vi "Zamojski_prac8.vi"() -> ()   [LabVIEW 2020]
uses:
  <vilib>/Platform/TimedLoop/XDataNode/timing_clust.ctl
  <vilib>/Platform/TimedLoop/XDataNode/nitl_modes.ctl
  <vilib>/Platform/TimedLoop/XDataNode/wakeup.ctl
  <vilib>/Platform/TimedLoop/scheduler/LVUserAPI/_suppVIs/Create_1kHz_TSource.vi
  <vilib>/platform/TimedLoop/XDataNode/XDataNode.xnode
  <vilib>/Platform/TimedLoop/XDataNode/XDNodeRunTimeDep.lvlib
panel:
  out "L2 Error":errorcluster
  out "czas_pocz_L1":dbl
  out "L1 Error":errorcluster
  out "L1 Iteracja":dbl
  out "L2 Koniec":bool
  out "L1 Koniec":bool
  out "L2 Stop":dbl
  out "L2 End":dbl
  out "L1 Stop":dbl
  out "L1 End":dbl
  out "L2 Iteracja":dbl
  out "SO End":dbl
  out "SO Start":dbl
  in  "Synchronizacja":bool
  in  "Okres (s)":dbl=0.5 min=0.5 max=20.0 step=0.5
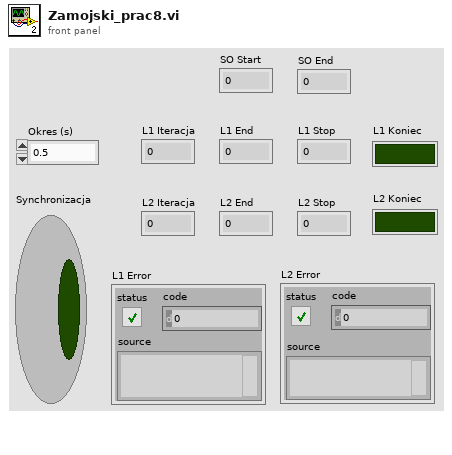
[diagram p1: front panel]
types:
  T1 = typedef "XDNodeRunTimeDep.lvlib/timing_clust.ctl" = cluster{"Expected End [f-1]":u64, "Actual End [f-1]":u64, "Finished Late? [f-1]":bool, "Expected End [i-1]":u64, "Actual End [i-1]":u64, "Finished Late? [i-1]":bool, "Expected Start [i]":u64, "Actual Start [i]":u64, "Expected Start [f]":u64, "Actual Start [f]":u64, "Source Name":string, "Structure Name":string, "Period":i64, "Deadline":i64, "Offset":i64, "Start":i64, "Priority":i32, "Timeout":i32, "Mode":T2, "Wakeup Reason":T3, "Error":errorcluster, "Source Type":string, "Secondary Source Type":string, "Global End Time":u64, "Global Start Time":u64, "Frame Duration":u64, "Iteration Duration":u64, "Assigned CPU":i32, "I/O Scan Engine Mode":u32}
  T2 = typedef "XDNodeRunTimeDep.lvlib/nitl_modes.ctl" = enum32{"No Change", "Process missed periods, maintain original phase", "Discard missed periods, maintain original phase", "Process missed periods, ignore original phase", "Discard missed periods, ignore original phase"}
  T3 = typedef "XDNodeRunTimeDep.lvlib/wakeup.ctl" = enum32{"Normal", "Aborted", "Asynchronous wakeup", "Timing source error", "Timed loop error", "Timeout"}
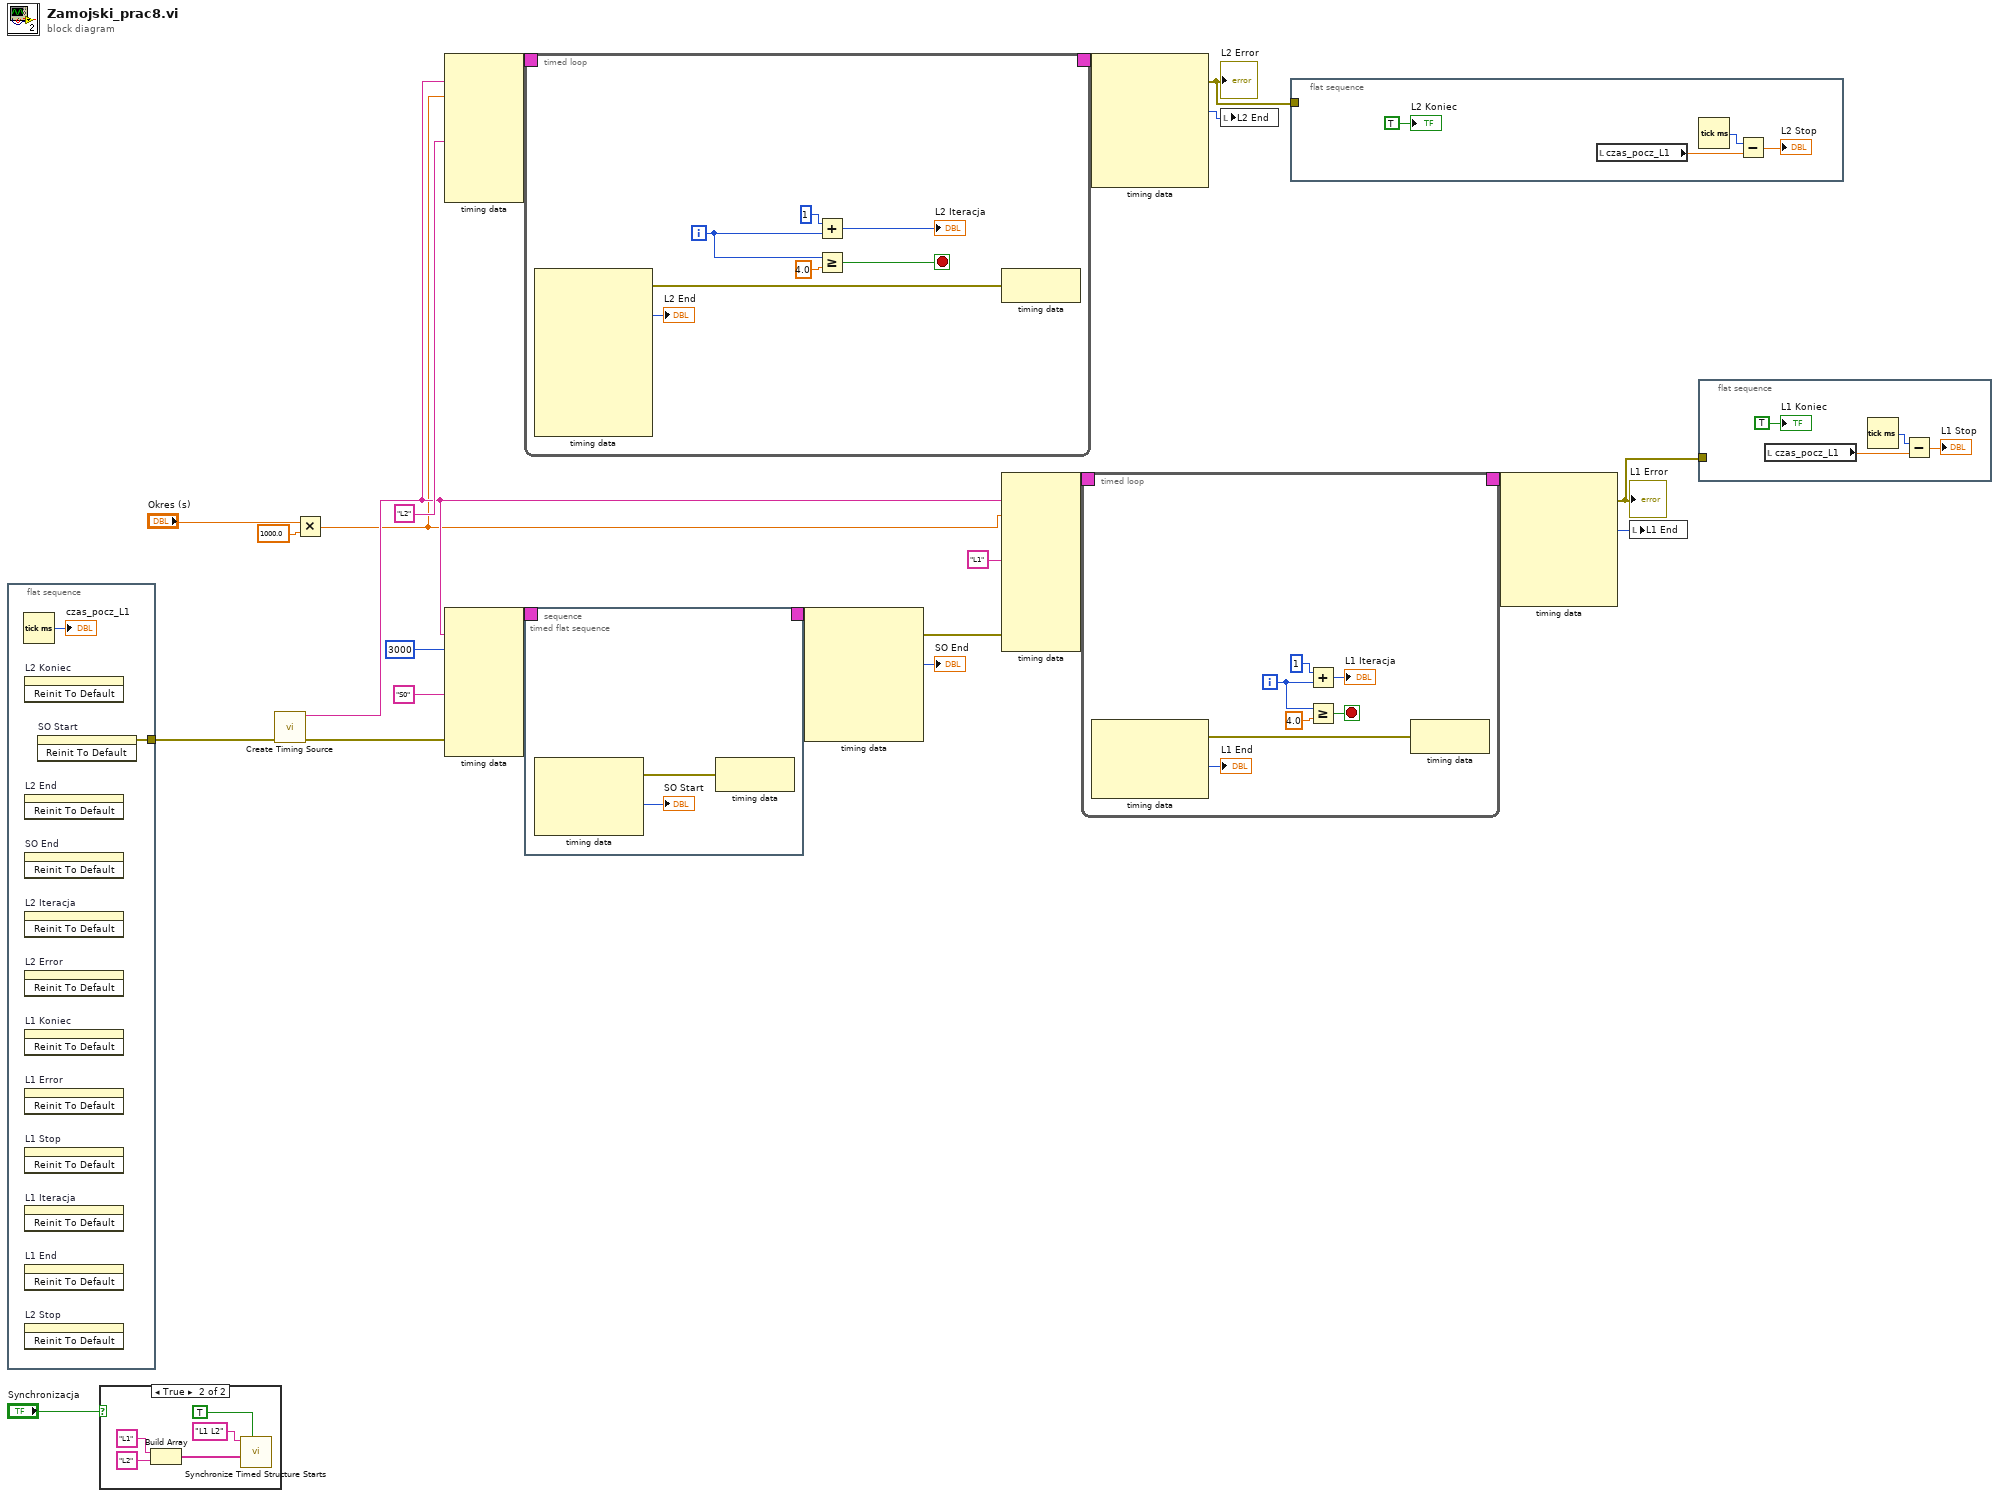
[diagram p0: block diagram]
diagram:
  n1 = flat-sequence {
    tunnel: [w24] -> w2
    frame #0 {
      n2 = Tick Count (ms)() -> (millisecond timer value=→"czas_pocz_L1":u32)
      n3 = invoke on="L2 Koniec" class="Bool (strict)" method="Reinit To Default"() -> ()  [unwired: 3 in, 3 out]
      n4 = invoke on="L2 End" class="DigNum (strict)" method="Reinit To Default"() -> ()  [unwired: 3 in, 3 out]
      n5 = invoke on="SO End" class="DigNum (strict)" method="Reinit To Default"() -> ()  [unwired: 3 in, 3 out]
      n6 = invoke on="L2 Iteracja" class="DigNum (strict)" method="Reinit To Default"() -> ()  [unwired: 3 in, 3 out]
      n7 = invoke on="L2 Error" class="Clust (strict)" method="Reinit To Default"() -> ()  [unwired: 3 in, 3 out]
      n8 = invoke on="L1 Koniec" class="Bool (strict)" method="Reinit To Default"() -> ()  [unwired: 3 in, 3 out]
      n9 = invoke on="L1 Error" class="Clust (strict)" method="Reinit To Default"() -> ()  [unwired: 3 in, 3 out]
      n10 = invoke on="L1 Stop" class="DigNum (strict)" method="Reinit To Default"() -> ()  [unwired: 3 in, 3 out]
      n11 = invoke on="L1 Iteracja" class="DigNum (strict)" method="Reinit To Default"() -> ()  [unwired: 3 in, 3 out]
      n12 = invoke on="L1 End" class="DigNum (strict)" method="Reinit To Default"() -> ()  [unwired: 3 in, 3 out]
      n13 = invoke on="L2 Stop" class="DigNum (strict)" method="Reinit To Default"() -> ()  [unwired: 3 in, 3 out]
      n14 = invoke on="SO Start" class="DigNum (strict)" method="Reinit To Default"() -> (error out=w24:errorcluster)  [unwired: 3 in, 2 out]
    }
  }
  n15 = case shown="True" "Synchronizacja" {
    frame False {
    }
    frame True {
      n16 = Build Array("L1", "L2" ("element")) -> (w26:string[])
      n17 = call <vilib>:"Synchronize Timed Structure Starts.vi"("replace (T)"=TRUE, "timed structure names"=w26, "synchronization group name"="L1 L2") -> ()  [unwired: 7 in, 2 out]
    }
  }
  n18 = call-poly <vilib>:"Create Timing Source.vi"("error in (no error)"=w2) -> ("error out"=w14:errorcluster, "name (out)"=w5:string)  [unwired: 9 in]
  n19 = Multiply(x="Okres (s)", y=1000.0) -> (x*y=w4:dbl)
  n20 = node-c288(w5, w4, "L2" ("Structure Name")) -> (w21:T1)  [unwired: 5 in]
  n21 = node-c288(w5, i64 3000 ("Offset"), "S0" ("Structure Name"), w14) -> (w17:T1)  [unwired: 4 in]
  n22 = timed-loop {
    timing: w21 -> [_]
    timing-out: [_] -> w20
    i -> [w31]
    stop <- w32 stop-if-true
    n23 = node-c288() -> (w37:errorcluster, →"L2 End":i64)  [unwired: 1 in, 8 out]
    n24 = Add(x=1, y=w31) -> (x+y=→"L2 Iteracja":i32)
    n25 = Greater Or Equal?(x=w31, y=4.0) -> (x >= y?=w32:bool)
    n26 = node-c288(w37) -> ()  [unwired: 1 out]
  }
  n27 = timed-sequence {
    timing: w17 -> [_]
    timing-out: [_] -> w16
    n28 = timed-flat-sequence {
      n29 = node-c288() -> (w45:errorcluster, →"SO Start":i64)  [unwired: 1 in, 2 out]
      n30 = node-c288(w45) -> ()  [unwired: 1 out]
    }
  }
  n31 = node-c288(w16) -> (w15:errorcluster, →"SO End":i64)  [unwired: 5 out]
  n32 = node-c288(w5, w4, "L1" ("Structure Name"), w15) -> (w23:T1)  [unwired: 6 in]
  n33 = timed-loop {
    timing: w23 -> [_]
    timing-out: [_] -> w22
    i -> [w55]
    stop <- w54 stop-if-true
    n34 = node-c288() -> (w58:errorcluster, →"L1 End":i64)  [unwired: 1 in, 2 out]
    n35 = Add(x=1, y=w55) -> (x+y=→"L1 Iteracja":i32)
    n36 = Greater Or Equal?(x=w55, y=4.0) -> (x >= y?=w54:bool)
    n37 = node-c288(w58) -> ()  [unwired: 1 out]
  }
  n38 = node-c288(w20) -> (w18:errorcluster, w3:i64)  [unwired: 5 out]
  "L2 Error" <- w18
  n39 = local write "L2 End"(w3) -> ()
  n40 = flat-sequence {
    tunnel: w18 -> [_]
    frame #0 {
      n41 = local read "czas_pocz_L1"() -> (w67:dbl)
      n42 = Tick Count (ms)() -> (millisecond timer value=w66:u32)
      n43 = Subtract(x=w66, y=w67) -> (x-y=→"L2 Stop":dbl)
      "L2 Koniec" <- TRUE ("L2 Koniec")
    }
  }
  n44 = node-c288(w22) -> (w19:errorcluster, w7:i64)  [unwired: 5 out]
  "L1 Error" <- w19
  n45 = local write "L1 End"(w7) -> ()
  n46 = flat-sequence {
    tunnel: w19 -> [_]
    frame #0 {
      n47 = local read "czas_pocz_L1"() -> (w69:dbl)
      n48 = Tick Count (ms)() -> (millisecond timer value=w71:u32)
      n49 = Subtract(x=w71, y=w69) -> (x-y=→"L1 Stop":dbl)
      "L1 Koniec" <- TRUE ("L1 Koniec")
    }
  }
